vi "Load and Check Tach Wave File.vi"(6 "check?":bool, 8 "error in (no error)":bool, 9 "check sum":i16[](array[numeric]), 10 "file names":string[](array[string]), 11 "wave file path in":path) -> (0 "error out":bool, 1 "sample rate":u32, 2 "tach data":i16[](array[numeric]), 3 "wave file path out":path)   [LabVIEW 2017]
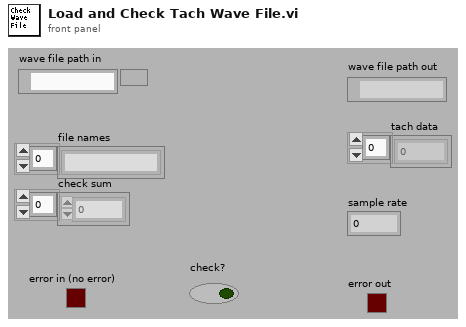
[diagram p1: front panel]
types:
  T1 = typedef "Sound Format+.ctl" = cluster{"quality":enum16{"mono", "stereo"}, "sample rate":u32, "bits/sample":enum16{"8 bit", "16 bit"}}
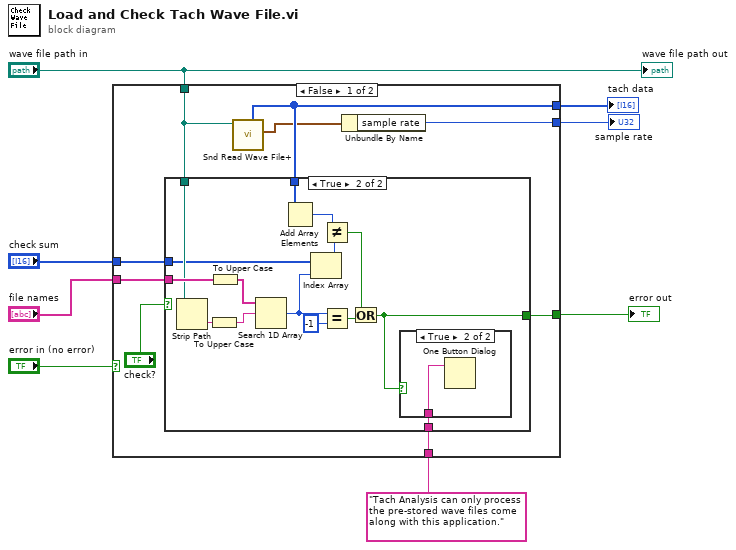
[diagram p0: block diagram]
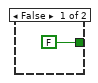
[diagram p2: hidden frame]
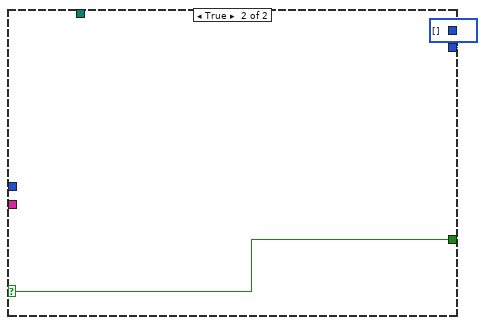
[diagram p4: hidden frame]
diagram:
  n1 = case shown="False" "error in (no error)" {
    selector: "error in (no error)" -> [_ w37]
    tunnel: [w10 w37] -> w8
    tunnel: "wave file path in" -> [w16 _]
    tunnel: "file names" -> [w17 _]
    tunnel: [w15 i16[] [] ("mono 16-bit")] -> w4
    tunnel: "check sum" -> [w14 _]
    tunnel: [w12 u32 1 ("sample rate")] -> w2
    tunnel: "Tach Analysis can only process the pre-stored wave files come along with this application." -> [w11 _]
    frame False {
      n2 = call <vilib>:"Snd Read Wave File+.vi"("wave file path"=w16) -> ("sound format"=w13:T1, "mono 16-bit"=w15:i16[])  [unwired: 4 in, 5 out]
      n3 = case shown="True" "check?" {
        tunnel: w17 -> [_ w32]
        tunnel: w16 -> [_ w30]
        tunnel: w15 -> [_ w29]
        tunnel: w14 -> [_ w26]
        tunnel: w11 -> [_ w20]
        tunnel: [FALSE w19] -> w10
        frame False {
        }
        frame True {
          n4 = Strip Path(path=w30) -> (name=w33:string)  [unwired: 1 out]
          n5 = To Upper Case(1:w33) -> (0:w31:string)
          n6 = To Upper Case(1:w32) -> (0:w24:string[])
          n7 = Search 1D Array(1D array=w24, element=w31) -> (index of element=w21:i32)  [unwired: 1 in]
          n8 = Add Array Elements(numeric array=w29) -> (sum=w27:i16)
          n9 = Index Array(array=w26, index=w21) -> (element=w25:i16)
          n10 = Not Equal?(x=w27, y=w25) -> (x != y?=w22:bool)
          n11 = Equal?(x=w21, y=-1) -> (x = y?=w28:bool)
          n12 = Or(x=w22, y=w28) -> (x .or. y?=w19:bool)
          n13 = case shown="True" w19 {
            tunnel: w20 -> [_ w34]
            frame False {
            }
            frame True {
              n14 = One Button Dialog(message=w34) -> ()  [unwired: 1 in, 1 out]
            }
          }
        }
      }
      n15 = Unbundle By Name(w13) -> ("sample rate"=w12:u32)
    }
    frame True {
    }
  }
  "error out" <- w8
  "tach data" <- w4
  "sample rate" <- w2
  "wave file path out" <- "wave file path in"
